vi "系统设置_总磷.vi"() -> ()   [LabVIEW 2016]
uses:
  <vilib>/Utility/miscctls.llb/LVPointTypeDef.ctl
  <vilib>/Utility/config.llb/Read Key (Boolean).vi
  <vilib>/Utility/config.llb/Write Key (Boolean).vi
  <vilib>/ptbypt/NI_PtbyPt.lvlib
  <vilib>/Utility/config.llb/NI_LVConfig.lvlib
panel:
  in  "周期启动":bool
  in  "24H周期设置":T1(xcontrol)
  # "s"
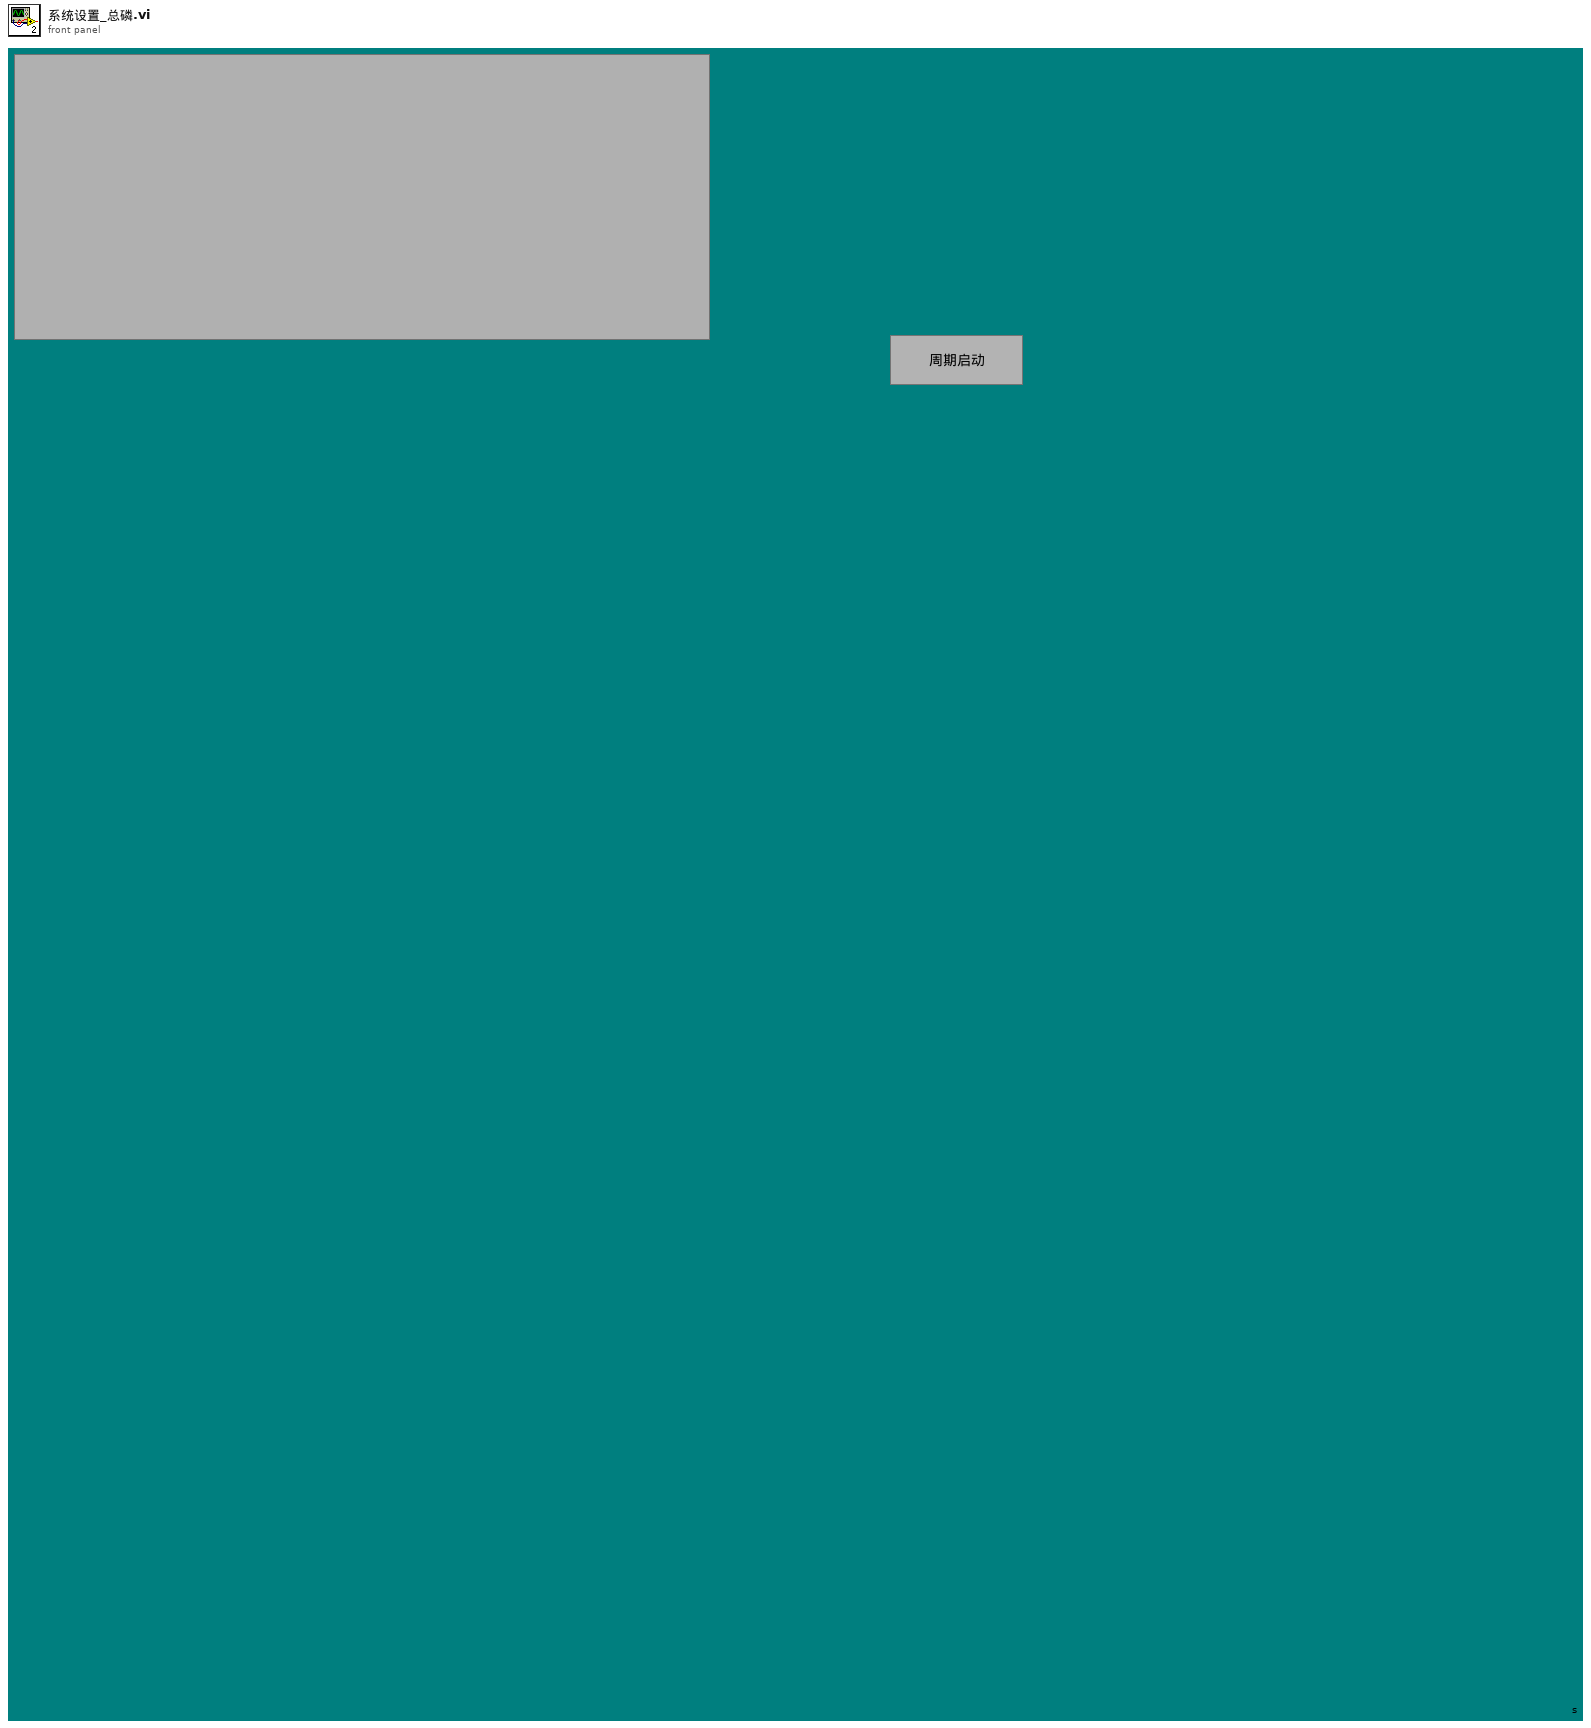
[diagram p1: front panel]
types:
  T1 = cluster{"00H":bool, "01H":bool, "02H":bool, "03H":bool, "04H":bool, "05H":bool, "06H":bool, "07H":bool, "08H":bool, "09H":bool, "10H":bool, "11H":bool, "12H":bool, "13H":bool, "14H":bool, "15H":bool, "16H":bool, "17H":bool, "18H":bool, "19H":bool, "20H":bool, "21H":bool, "22H":bool, "23H":bool}
  T2 = cluster{"记录类型":enum16{"操作日志", "报警信息"}, "记录设备":string, "记录内容":string}
  T3 = typedef "LVPointTypeDef.ctl" = cluster{"Horizontal":i16, "Vertical":i16}
  T4 = cluster{"站号":u16, "量程切换":enum32{"H", "L", "AUTO"}, "控制命令":enum16{"启动测量", "标样核查", "零点核查", "跨度核查", "空白测试", "平行样测试", "加标回收", "空白校准", "标样校准", "初始化（清洗）", "停止测试", "仪器重启", "校时", "模式设置", "测量间隔设置", "盲样测试"}, "模式设置":enum16{"待机", "连续模式", "周期模式", "定点模式", "受控模式", "手动模式"}, "测量间隔":u16}
  T5 = cluster{"记录类型":enum16{"操作日志", "报警信息"}, "记录内容":string, "记录内容 2":string}
  T6 = typedef "NI_LVConfig.lvlib/Config Data RefNum.ctl" = refnum<k1>
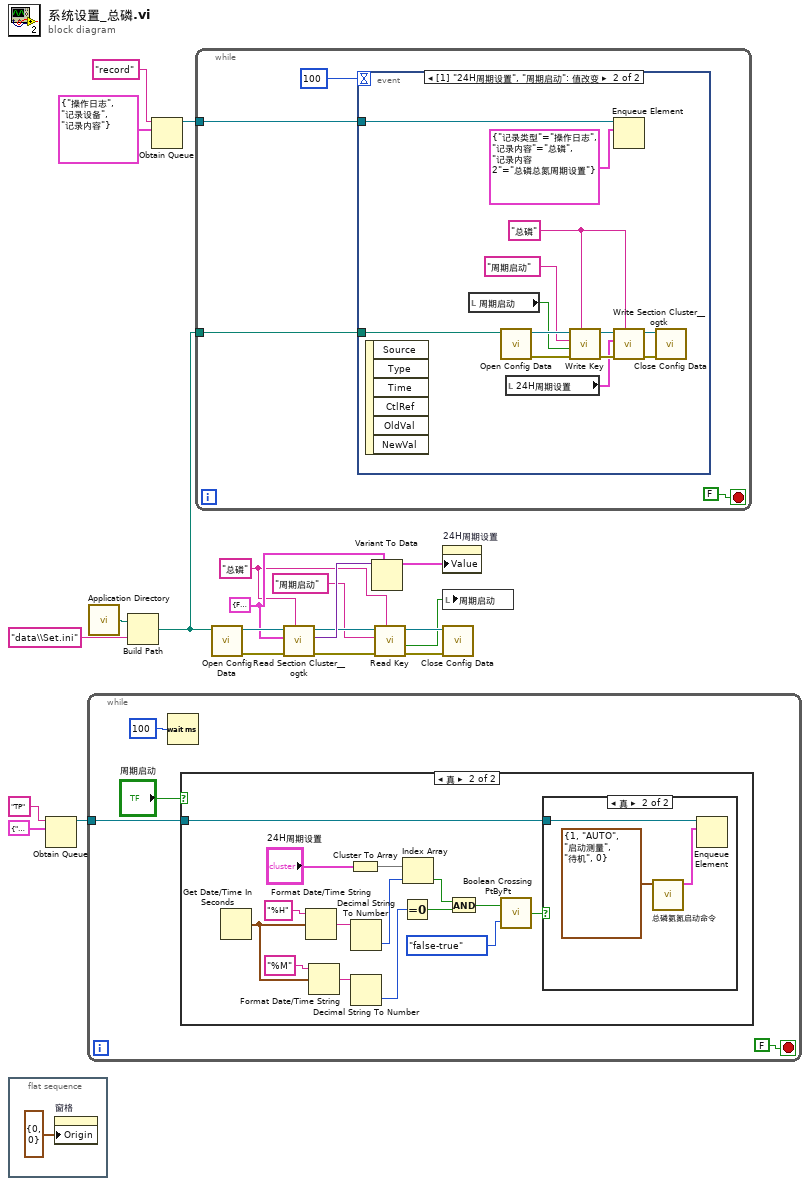
[diagram p0: block diagram]
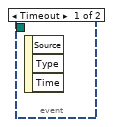
[diagram p4: hidden frame]
diagram:
  w8 = "总磷" ("section")
  w16 = T1 {"00H"=FALSE, "01H"=FALSE, "02H"=FALSE, "03H"=FALSE, "04H"=FALSE, "05H"=FALSE, "06H"=FALSE, "07H"=FALSE, "08H"=FALSE, "09H"=FALSE, "10H"=FALSE, "11H"=FALSE, "12H"=FALSE, "13H"=FALSE, "14H"=FALSE, "15H"=FALSE, "16H"=FALSE, "17H"=FALSE, "18H"=FALSE, "19H"=FALSE, "20H"=FALSE, "21H"=FALSE, "22H"=FALSE, "23H"=FALSE} ("24H周期设置")
  n1 = flat-sequence {
    frame #0 {
      n2 = property on="窗格" class="Pane"("Origin"=T3 {"Horizontal"=0, "Vertical"=0} ("原点")) -> ()  [unwired: 2 in, 2 out]
    }
  }
  n3 = Obtain Queue(name (unnamed)="TP" ("名称（未命名）"), element data type=cluster{"命令":string, "data":variant} {"命令"="", "data"=variant}) -> (queue out=w1:refnum<queue>)  [unwired: 3 in, 2 out]
  n4 = while {
    tunnel: w1 -> [w23]
    stop <- FALSE stop-if-true
    n5 = Wait (ms)(milliseconds to wait=u32 100 ("等待时间（毫秒）")) -> ()  [unwired: 1 out]
    n6 = case shown="真" "周期启动" {
      tunnel: w23 -> [_ w27]
      frame False {
      }
      frame True {
        n7 = Get Date/Time In Seconds() -> (seconds since 1Jan1904=w40:timestamp)
        n8 = Format Date/Time String(time format string (%c)="%H" ("时间格式字符串(%c)"), seconds (now)=w40) -> (date/time string=w36:string)  [unwired: 1 in]
        n9 = Format Date/Time String(time format string (%c)="%M" ("时间格式字符串(%c)"), seconds (now)=w40) -> (date/time string=w34:string)  [unwired: 1 in]
        n10 = Cluster To Array(cluster="24H周期设置") -> (array=w37:bool[])
        n11 = Decimal String To Number(string=w36) -> (number=w35:i32)  [unwired: 2 in, 1 out]
        n12 = Decimal String To Number(string=w34) -> (number=w33:i32)  [unwired: 2 in, 1 out]
        n13 = Equal To 0?(x=w33) -> (x = 0?=w31:bool)
        n14 = Index Array(array=w37, index=w35) -> (element=w32:bool)
        n15 = And(x=w32, y=w31) -> (x .and. y?=w30:bool)
        n16 = call <vilib>:"Boolean Crossing PtByPt.vi"("direction"=enum16{"either", "false-true", "true-false"}."false-true", "input"=w30) -> ("crossing"=w28:bool)  [unwired: 1 in]
        n17 = case shown="真" w28 {
          tunnel: w27 -> [_ w42]
          frame False {
          }
          frame True {
            n18 = call "总磷氨氮启动命令.vi"("参数"=T4 {"站号"=1, "量程切换"=enum."AUTO", "控制命令"=enum."启动测量", "模式设置"=enum."待机", "测量间隔"=0}) -> ("启动命令"=w44:cluster{"命令":string, "data":variant})  [unwired: 10 in]
            n19 = Enqueue Element(queue=w42, element=w44) -> ()  [unwired: 2 in, 3 out]
          }
        }
      }
    }
  }
  n20 = call <vilib>:"Application Directory.vi"() -> ("Application Directory"=w20:path)
  n21 = Build Path(base path=w20, name or relative path="data\\Set.ini" ("名称或相对路径")) -> (appended path=w10:path)
  n22 = Obtain Queue(name (unnamed)="record" ("名称（未命名）"), element data type=T2 {"记录类型"=enum."操作日志", "记录设备"="记录设备", "记录内容"="记录内容"}) -> (queue out=w5:refnum<queue>)  [unwired: 3 in, 2 out]
  n23 = while {
    tunnel: w10 -> [w46]
    tunnel: w5 -> [w45]
    stop <- FALSE stop-if-true
    n24 = event shown="[1] \"24H周期设置\", \"周期启动\": 值改变" {
      selector: _ -> [_ _]
      dyn-events: _ -> [_ _]
      timeout: 100 -> [_ _]
      tunnel: w46 -> [_ w51]
      tunnel: w45 -> [_ w50]
      event Timeout {
        n25 = event-data() -> ()  [unwired: 1 in, 3 out]
      }
      event "24H周期设置", "周期启动": Value Change {
        w55 = "总磷" ("section")
        n26 = event-data() -> ()  [unwired: 1 in, 6 out]
        n27 = local read "周期启动"() -> (w53:bool)
        n28 = call <vilib>:"Open Config Data.vi"("configuration file path"=w51) -> ("error out"=w60:errorcluster, "refnum"=w61:T6)  [unwired: 8 in, 1 out]
        n29 = local read "24H周期设置"() -> (w52:T1)
        n30 = call-poly <vilib>:"Write Key.vi"("section"=w55, "error in (no error)"=w60, "value"=w53, "key"="周期启动", "refnum"=w61) -> ("error out"=w58:errorcluster, "refnum out"=w59:T6)  [unwired: 4 in, 1 out]
        n31 = Enqueue Element(queue=w50, element=T5 {"记录类型"=enum."操作日志", "记录内容"="总磷", "记录内容 2"="总磷总氮周期设置"} ("元素")) -> ()  [unwired: 2 in, 3 out]
        n32 = call <userlib>:"Write Section Cluster__ogtk.vi"("section (optional)"=w55, "error in (no error)"=w58, "Section Formatted Cluster"=w52, "refnum"=w59) -> ("error out"=w56:errorcluster, "dup refnum"=w57:T6)  [unwired: 6 in]
        n33 = call <vilib>:"Close Config Data.vi"("error in (no error)"=w56, "refnum"=w57) -> ()  [unwired: 8 in, 2 out]
      }
    }
  }
  n34 = call <vilib>:"Open Config Data.vi"("configuration file path"=w10) -> ("error out"=w18:errorcluster, "refnum"=w19:T6)  [unwired: 8 in, 1 out]
  n35 = call <userlib>:"Read Section Cluster__ogtk.vi"("section (optional)"=w8, "error in (no error)"=w18, "Section Formatted Cluster Type"=w16, "refnum"=w19) -> ("error out"=w14:errorcluster, "Section Formatted Cluster"=w17:variant, "dup refnum"=w15:T6)  [unwired: 3 in, 2 out]
  n36 = Variant To Data(type=w16, Variant=w17) -> (data=w9:T1)  [unwired: 1 in, 1 out]
  n37 = call-poly <vilib>:"Read Key.vi"("section"=w8, "error in (no error)"=w14, "key"="周期启动", "refnum"=w15) -> ("error out"=w12:errorcluster, "value"=w7:bool, "refnum out"=w13:T6)  [unwired: 4 in, 1 out]
  n38 = property on="24H周期设置" class="24H周期设置 (严格)"("Value"=w9) -> ()  [unwired: 2 in, 2 out]
  n39 = local write "周期启动"(w7) -> ()
  n40 = call <vilib>:"Close Config Data.vi"("error in (no error)"=w12, "refnum"=w13) -> ()  [unwired: 8 in, 2 out]
